vi "Read readInitialTime.vi"(8 "error in (no error)":errorcluster, 11 "State in":refnum<class "ElectrometerState.lvclass">) -> (0 "error out":errorcluster, 2 "readInitialTime":dbl, 3 "State out":refnum<class "ElectrometerState.lvclass">)   [LabVIEW 2016, in "ElectrometerState.lvclass"]
uses:
  ElectrometerState.lvclass
  ElectrometerState.lvclass/ElectrometerState.ctl
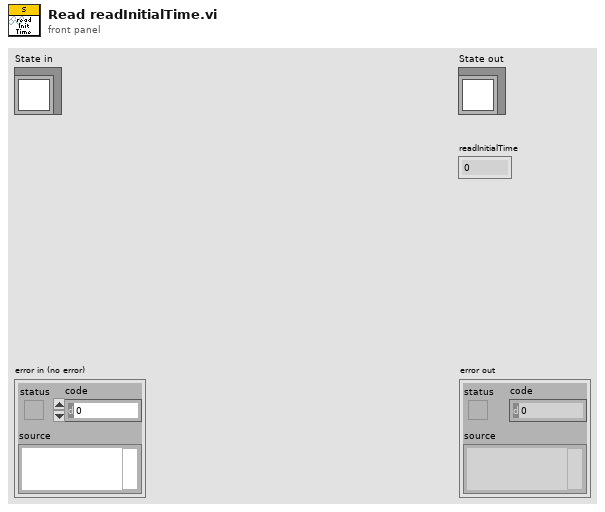
[diagram p1: front panel]
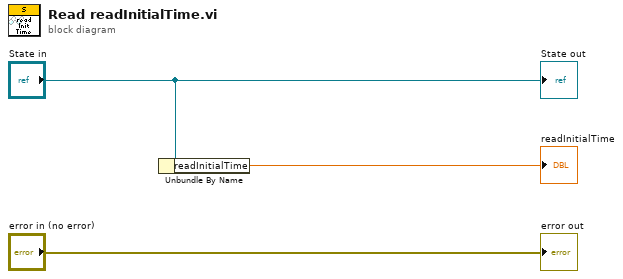
[diagram p0: block diagram]
diagram:
  n1 = Unbundle By Name("State in") -> ("readInitialTime"=→"readInitialTime":dbl)
  "error out" <- "error in (no error)"
  "State out" <- "State in"
